vi "AddPointToPath.vi"(8 "error in":T1, 10 "CoordY":sgl format="%#_g µm", 11 "CoordX":sgl format="%#_g µm") -> (0 "error out":T1, 3 "Cluster":cluster{"CoordX":sgl, "CoordY":sgl} {"CoordX" format="%#_g µm"; "CoordY" format="%#_g µm"})   [LabVIEW 2016]
doc: "Adds a point specified by its coordinates (relative to the scanning start point) to the pathmode list."
uses:
  Controls/Error_Out.ctl
  Files_ASC500/DLL/ASC500_RemoteControlV27.dll
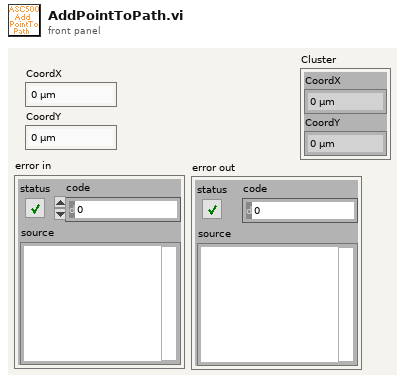
[diagram p1: front panel]
types:
  T1 = typedef "Error_Out.ctl" = errorcluster
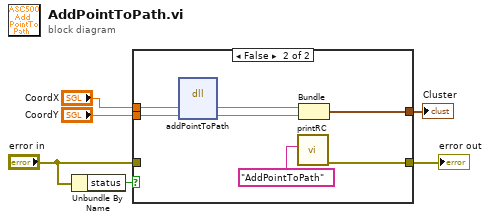
[diagram p0: block diagram]
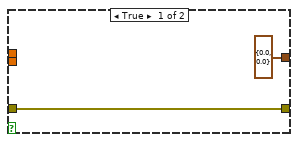
[diagram p2: hidden frame]
diagram:
  n1 = Unbundle By Name("error in") -> ("status"=w6:bool)
  n2 = case shown="False" w6 {
    tunnel: "error in" -> [w8 _]
    tunnel: [w8 w14] -> w4
    tunnel: "CoordX" -> [_ w13]
    tunnel: "CoordY" -> [_ w12]
    tunnel: [cluster{"CoordX":sgl, "CoordY":sgl} {"CoordX"=0.0, "CoordY"=0.0} w9] -> w1
    frame True {
    }
    frame False {
      n3 = dll-call lib="G:/SCMOperations/Share/ELE/Produkt Information/ASC500/04 Remote Control/02 development versions/2018Nov06/Files_ASC500/DLL/ASC500_RemoteControlV27.dll" fn="addPointToPath"("CoordX"=w13, "CoordY"=w12) -> ("CoordX"=w11:sgl, "CoordY"=w10:sgl)  [unwired: 4 in, 2 out]
      n4 = call "printRC.vi"("additional information"="AddPointToPath") -> ("error out"=w14:T1)  [unwired: 10 in]
      n5 = Bundle("CoordX"=w11, "CoordY"=w10) -> (w9:cluster{"CoordX":sgl, "CoordY":sgl})  [unwired: 1 in]
    }
  }
  "error out" <- w4
  "Cluster" <- w1
